vi "PVC_Copper_Barrel.vi"(0 "Wm":dbl, 5 "Hm":dbl, 7 "R":dbl, 9 "Cos_net":dbl, 11 "Sin_net":dbl) -> (4 "height":dbl)   [LabVIEW 2019, in "Algorithm.lvclass"]
uses:
  FrameworkOverrides/Algorithm.lvclass
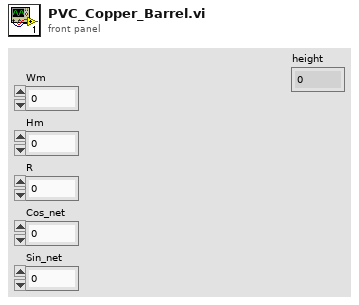
[diagram p1: front panel]
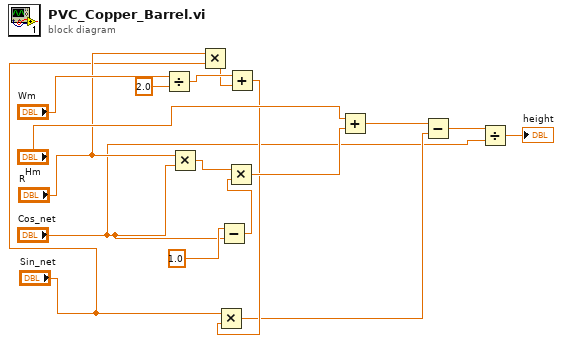
[diagram p0: block diagram]
diagram:
  n1 = Divide(x="Wm", y=2.0) -> (x/y=w9:dbl)
  n2 = Multiply(x="R", y="Cos_net") -> (x*y=w17:dbl)
  n3 = Multiply(x="R", y="Sin_net") -> (x*y=w6:dbl)
  n4 = Subtract(x=1.0, y="Cos_net") -> (x-y=w15:dbl)
  n5 = Multiply(x=w17, y=w15) -> (x*y=w13:dbl)
  n6 = Add(x=w9, y=w6) -> (x+y=w5:dbl)
  n7 = Multiply(x="Sin_net", y=w5) -> (x*y=w4:dbl)
  n8 = Add(x="Hm", y=w13) -> (x+y=w12:dbl)
  n9 = Subtract(x=w12, y=w4) -> (x-y=w3:dbl)
  n10 = Divide(x=w3, y="Cos_net") -> (x/y=→"height":dbl)
